vi "Teleop.vi"(10 "Match Info":T1={"Autonomous Elapsed Seconds"=0.0, "TeleOp Elapsed Seconds"=0.0, "Disabled Elapsed Seconds"=0.0, "Visited Autonomous"=FALSE, "Visited TeleOp"=FALSE, "Visited Disabled"=FALSE, "Autonomous Settings"={"Autonomous Style"=enum."Independent", "VI Refnum"=refnum}}, 11 "Call Context":T2) -> ()   [LabVIEW 2015]
doc: "This VI is called for each TeleOp packet received from the DS where the robot is not disabled. It is often used to read from the joysticks and update I/O or to update setpoints for timed control loops. It should complete and return within 20 milliseconds or it may miss DS packets."
uses:
  <vilib>/Rock Robotics/WPI/DriverStation/WPI_DriverStationDerivedRobotMode.ctl
  <vilib>/Rock Robotics/WPI/DriverStation/WPI_DriverStationMatch Info.ctl
  <vilib>/Rock Robotics/WPI/Utilities/WPI_GetSetVariantRefNum.vi
  <vilib>/Rock Robotics/Network Tables/NT Write Boolean Array.vi
  <vilib>/Rock Robotics/Network Tables/NT Write Numeric Array.vi
  <vilib>/Rock Robotics/Network Tables/NT Read Boolean.vi
  <vilib>/Rock Robotics/Network Tables/NT Read Number.vi
  <vilib>/Rock Robotics/WPI/RobotDrive/WPI_RobotDriveArcadeDrive_Standard(NoSaturation).vi
  <vilib>/Rock Robotics/WPI/Ultrasonic/WPI_SonarMB1010AnalogRefNum Registry Get.vi
  <vilib>/Rock Robotics/WPI/Ultrasonic/WPI_SonarMB1010AnalogGetRange.vi
  <vilib>/Rock Robotics/Network Tables/NT Write Number.vi
panel:
  out "Cam Flip":string="Front"
  out "Cam angle\n compensation":dbl=180.0
  out "Drop":dbl=1.0
  out "stuff":dbl
  out "Distance":dbl
  out "Sample Slider 0":dbl(slide) scale=0.0..5.0
  out "Sample Boolean 1":bool
  out "Sample Boolean 0":bool
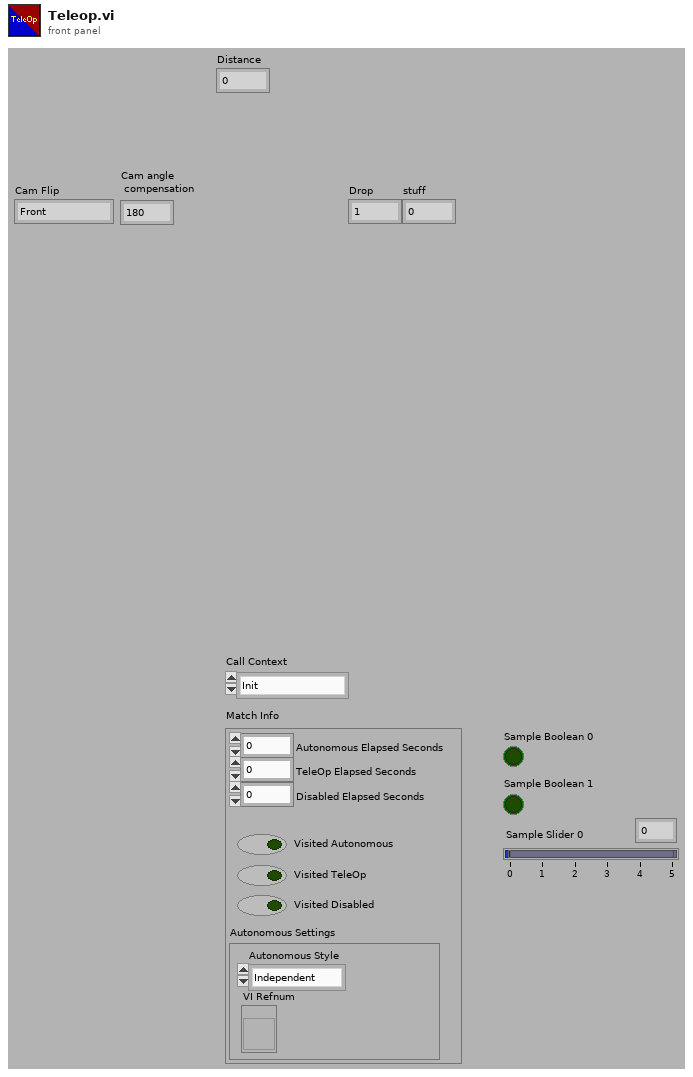
[diagram p1: front panel]
types:
  T1 = typedef "WPI_DriverStationMatch Info.ctl" = cluster{"Autonomous Elapsed Seconds":dbl, "TeleOp Elapsed Seconds":dbl, "Disabled Elapsed Seconds":dbl, "Visited Autonomous":bool, "Visited TeleOp":bool, "Visited Disabled":bool, "Autonomous Settings":cluster{"Autonomous Style":enum16{"Iterative", "Independent"}, "VI Refnum":refnum<vi>}}
  T2 = typedef "WPI_DriverStationDerivedRobotMode.ctl" = enum16{"Init", "Execute", "Stop"}
  T3 = typedef "WPI_JoystickDevRef.ctl" = cluster{"Device":T4}
  T4 = typedef "WPI_JoystickDeviceEnum.ctl" = enum16{"USB 0", "USB 1", "USB 2", "USB 3", "USB 4", "USB 5"}
  T5 = cluster{"Buttons[0]":bool, "Buttons[1]":bool, "Buttons[2]":bool, "Buttons[3]":bool, "Buttons[4]":bool, "Buttons[5]":bool, "Buttons[6]":bool, "Buttons[7]":bool, "Buttons[8]":bool}
  T6 = typedef "WPI_RobotDriveDevRef.ctl" = cluster{"DevStatus":errorcluster, "Motors[]":T7[], "Square Inputs":bool, "Max Output":dbl}
  T7 = typedef "WPI_MotorControlDeviceRef.ctl" = cluster{"DeviceStatus":errorcluster, "Type":T8, "PWM":cluster{"PWM Channel":T9, "DeadBand":T10}, "CAN":cluster{"Device Number":u8, "Control Mode":T11, "Semaphore":T12, "Max Vout":dbl, "TalonSRX Control Mode":T13}, "Invert":bool}
  T8 = typedef "WPI_MotorControlType.ctl" = enum16{"PWM", "CAN", "CANTalonSRX"}
  T9 = typedef "FPGA_DIOPWMChannel.ctl" = enum8{"PWM 0", "PWM 1", "PWM 2", "PWM 3", "PWM 4", "PWM 5", "PWM 6", "PWM 7", "PWM 8", "PWM 9", "PWM MXP 0", "PWM MXP 1", "PWM MXP 2", "PWM MXP 3", "PWM MXP 4", "PWM MXP 5", "PWM MXP 6", "PWM MXP 7", "PWM MXP 8", "PWM MXP 9", "Invalid"}
  T10 = typedef "WPI_PWMDeadband.ctl" = cluster{"Name":string, "maxPositivePwm":i32, "minPositivePwm":i32, "centerPwm":i32, "maxNegativePwm":i32, "minNegativePwm":i32, "angularRange":u16}
  T11 = typedef "WPI_CANJaguar_ControlMode.ctl" = enum8{"Percent VBus", "Current", "Speed", "Position", "Voltage"}
  T12 = typedef "Semaphore RefNum" = refnum<k1>
  T13 = typedef "WPI_CANTalonSRX_APIControlMode.ctl" = enum8{"Percent VBus", "Speed", "Position", "Slave", "Unchanged / Invalid", "Voltage Compensation", "Current", "Motion Profile"}
  T14 = typedef "WPI_ServoDeviceRef.ctl" = cluster{"DeviceStatus":errorcluster, "PWM Channel":T9, "DeadBand":T10}
  T15 = typedef "WPI_SonarMB1010AnalogDeviceRef.ctl" = cluster{"AIDeviceRef":T16, "Scaling factor (V/in)":dbl, "Average Bits":u8}
  T16 = typedef "WPI_AnalogChannelDevRef.ctl" = cluster{"DevStatus":errorcluster, "Analog Channel":T17}
  T17 = typedef "FPGA_AIChannel.ctl" = enum8{"AI 0", "AI 1", "AI 2", "AI 3", "AI MXP 0", "AI MXP 1", "AI MXP 2", "AI MXP 3", "Invalid"}
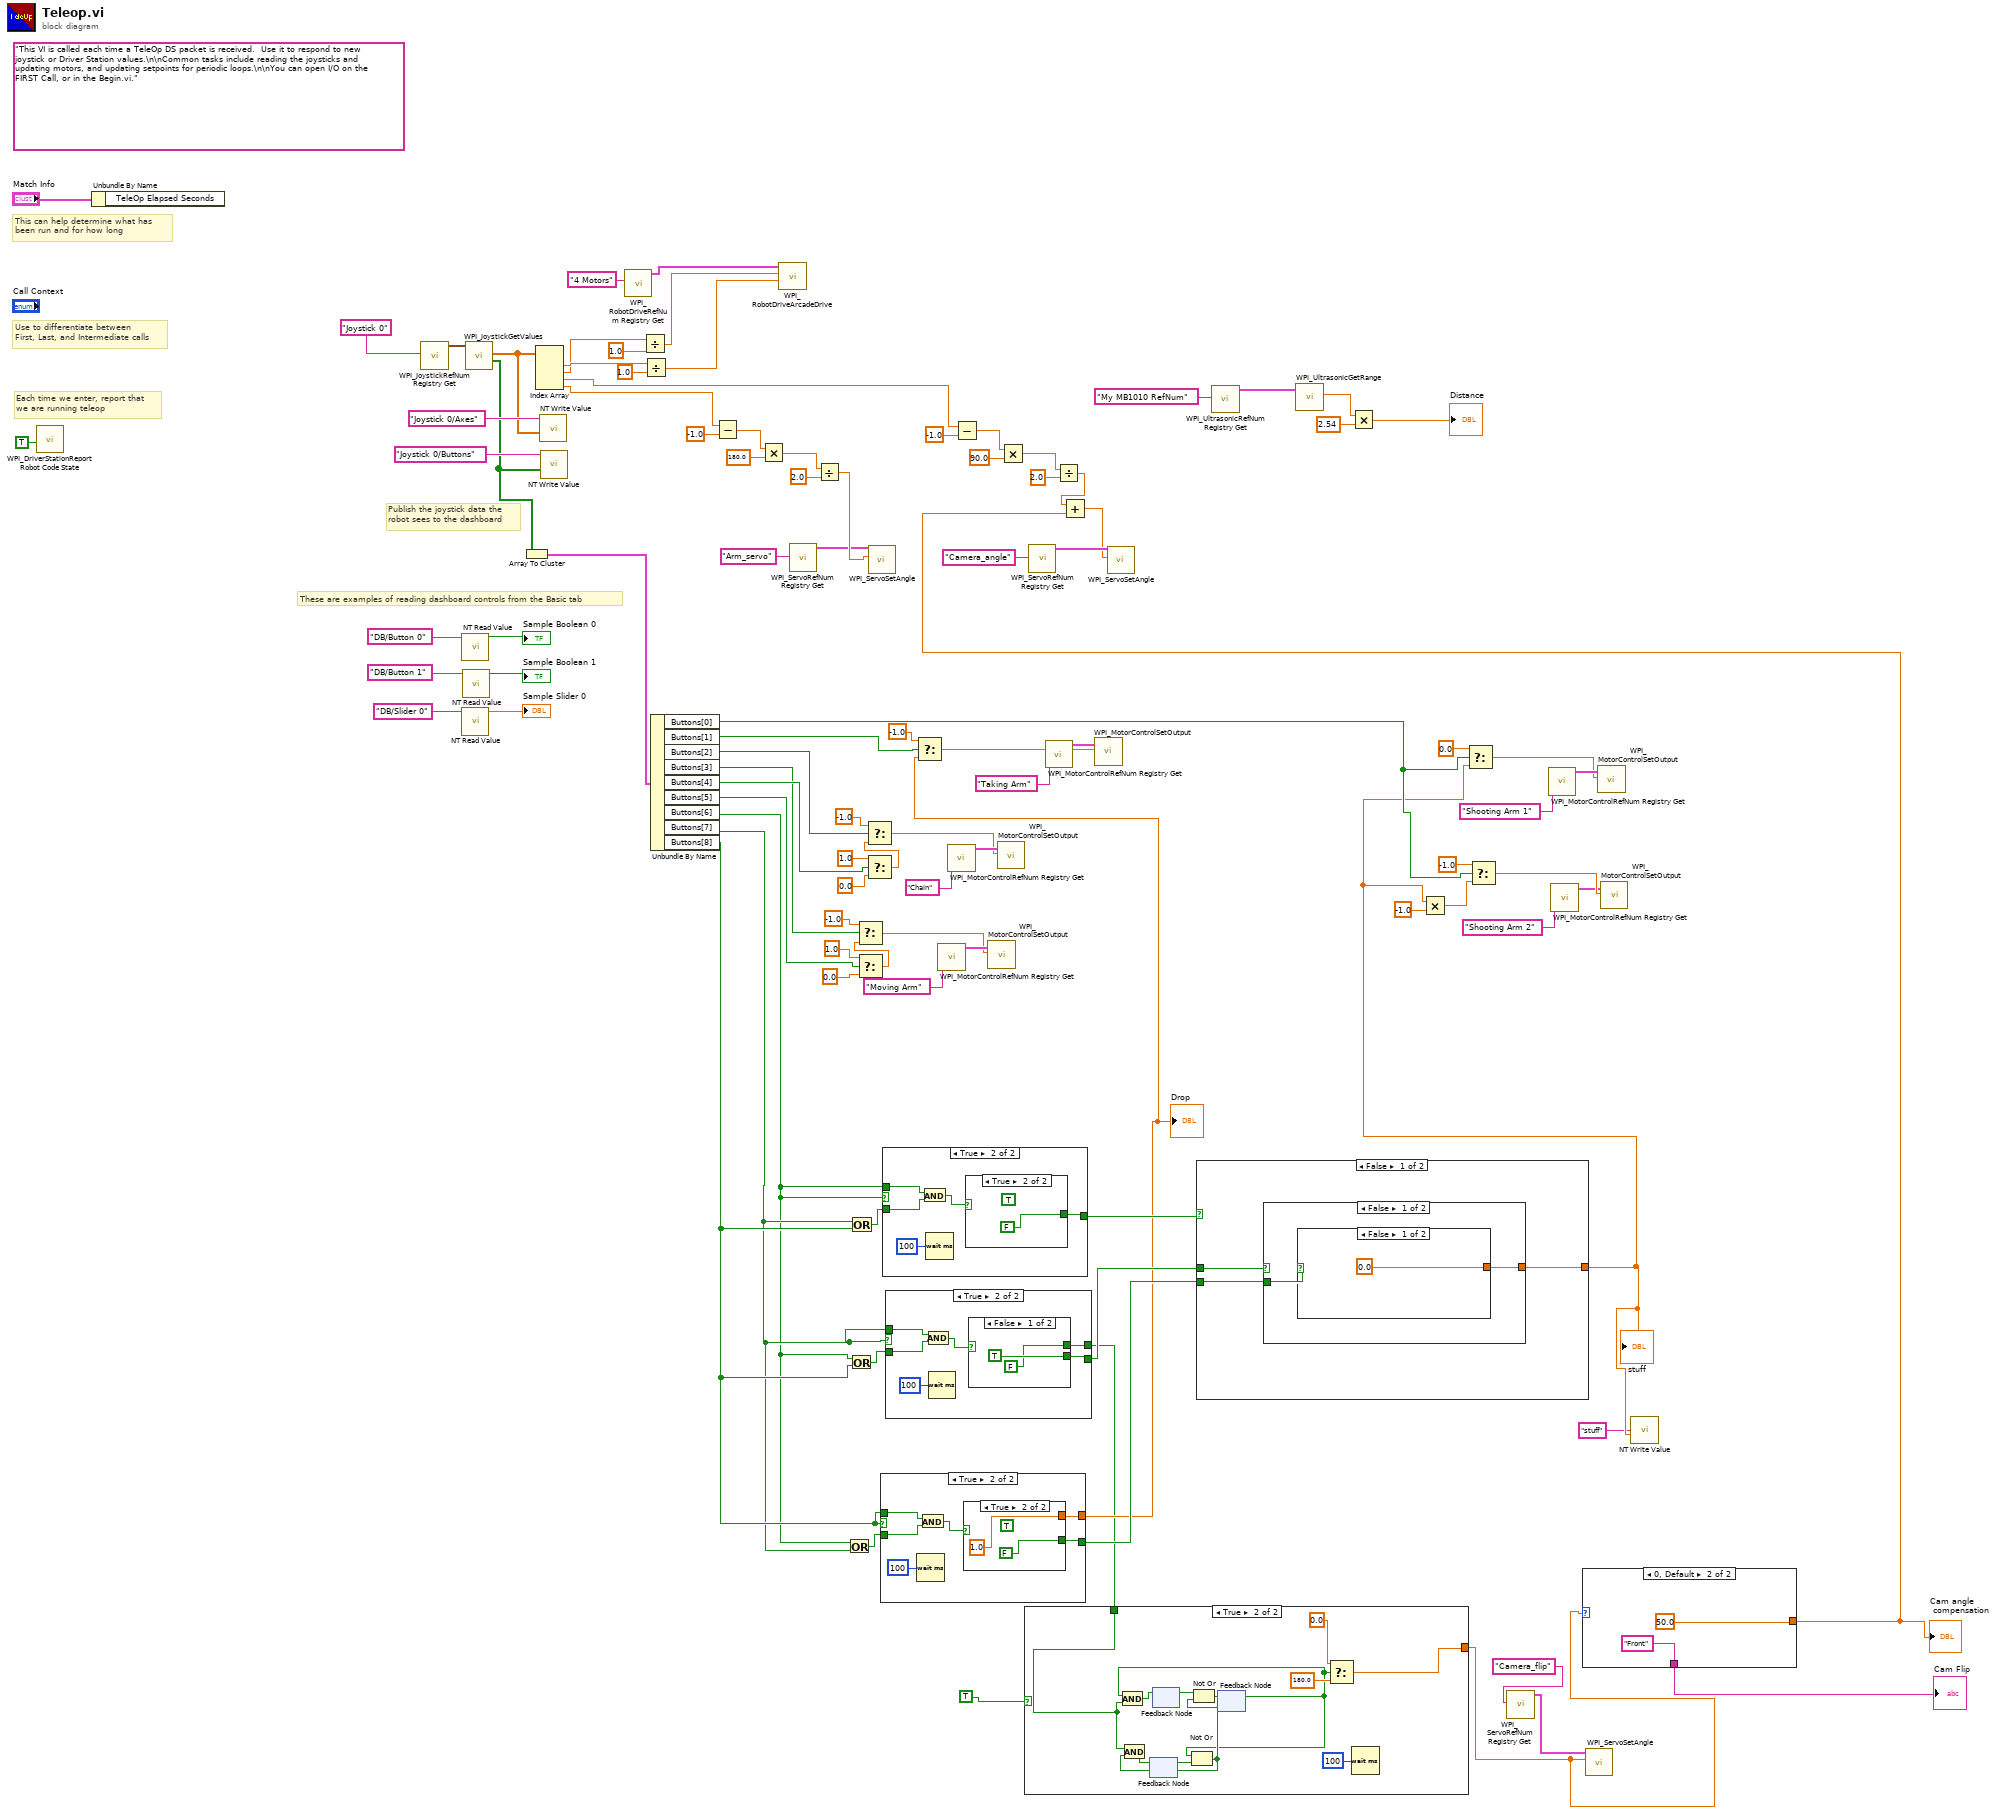
[diagram p0: block diagram]
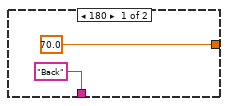
[diagram p2: hidden frame]
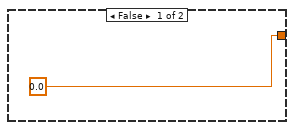
[diagram p3: hidden frame]
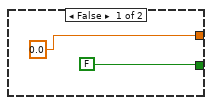
[diagram p4: hidden frame]
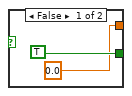
[diagram p5: hidden frame]
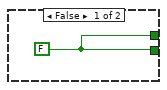
[diagram p6: hidden frame]
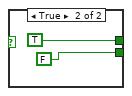
[diagram p7: hidden frame]
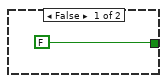
[diagram p8: hidden frame]
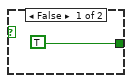
[diagram p9: hidden frame]
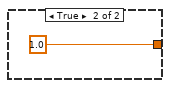
[diagram p10: hidden frame]
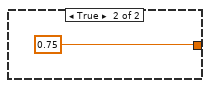
[diagram p11: hidden frame]
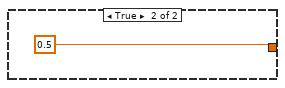
[diagram p12: hidden frame]
diagram:
  (unwired) "This VI is called each time a TeleOp DS packet is received.  Use it to respond to new joystick or Driver Station values.\n\nCommon tasks include reading the joysticks and updating motors, and updating setpoints for periodic loops.\n\nYou can open I/O on the FIRST Call, or in the Begin.vi."
  # "These are examples of reading dashboard controls from the Basic tab"
  # "Publish the joystick data the\nrobot sees to the dashboard"
  # "Each time we enter, report that\nwe are running teleop"
  # "Use to differentiate between\nFirst, Last, and Intermediate calls"
  # "This can help determine what has\nbeen run and for how long"
  n1 = call <vilib>:"WPI_DriverStationReport Robot Code State.vi"("TeleOp"=TRUE ("Autonomous")) -> ()  [unwired: 10 in, 1 out]
  n2 = Unbundle By Name("Match Info") -> ()  [unwired: 1 out]
  n3 = call <vilib>:"WPI_JoystickRefNum Registry Get.vi"("refnum name"="Joystick 0") -> ("JoystickDevRef"=w98:T3)  [unwired: 1 in, 9 out]
  n4 = call-poly <vilib>:"NT Read Value.vi"("Name"="DB/Button 0" ("refnum name")) -> ("Boolean"=→"Sample Boolean 0":bool)  [unwired: 9 in, 1 out]
  n5 = call-poly <vilib>:"NT Read Value.vi"("Name"="DB/Slider 0" ("refnum name")) -> ("Numeric"=→"Sample Slider 0":dbl)  [unwired: 9 in, 1 out]
  n6 = call-poly <vilib>:"NT Read Value.vi"("Name"="DB/Button 1" ("refnum name")) -> ("Boolean"=→"Sample Boolean 1":bool)  [unwired: 9 in, 1 out]
  n7 = call <vilib>:"WPI_JoystickGetValues.vi"("JoystickDevRef"=w98) -> ("Buttons"=w88:bool[], "Axes"=w87:dbl[])  [unwired: 6 in, 3 out]
  n8 = Array To Cluster(array=w88) -> (cluster=w42:T5)
  n9 = Index Array(array=w87) -> (element #1=w84:dbl, element #2=w83:dbl, element #3=w8:dbl, element #4=w16:dbl)  [unwired: 4 in]
  n10 = call-poly <vilib>:"NT Write Value.vi"("Numeric Array"=w87, "Name"="Joystick 0/Axes") -> ()  [unwired: 9 in, 1 out]
  n11 = call-poly <vilib>:"NT Write Value.vi"("Boolean Array"=w88, "Name"="Joystick 0/Buttons") -> ()  [unwired: 9 in, 1 out]
  n12 = call <vilib>:"WPI_RobotDriveRefNum Registry Get.vi"("refnum name"="4 Motors") -> ("RobotDriveDevRef"=w85:T6)  [unwired: 9 in, 1 out]
  n13 = Divide(x=w83, y=1.0) -> (x/y=w80:dbl)
  n14 = Divide(x=w84, y=1.0) -> (x/y=w79:dbl)
  n15 = Unbundle By Name "Unbundle By Name"(w42) -> ("Buttons[0]"=w55:bool, "Buttons[1]"=w43:bool, "Buttons[2]"=w47:bool, "Buttons[3]"=w45:bool, "Buttons[4]"=w46:bool, "Buttons[5]"=w44:bool, "Buttons[6]"=w22:bool, "Buttons[7]"=w23:bool, "Buttons[8]"=w25:bool)
  n16 = Subtract(x=w16, y=-1.0) -> (x-y=w35:dbl)
  n17 = Multiply(x=w35, y=180.0) -> (x*y=w37:dbl)
  n18 = call-poly <vilib>:"WPI_RobotDriveArcadeDrive.vi"("Y axis value"=w79, "X axis value"=w80, "RobotDriveDevRef"=w85) -> ()  [unwired: 6 in, 3 out]
  n19 = call <vilib>:"WPI_ServoRefNum Registry Get.vi"("refnum name"="Arm_servo") -> ("ServoDeviceRef"=w31:T14)  [unwired: 9 in, 1 out]
  n20 = Divide(x=w37, y=2.0) -> (x/y=w38:dbl)
  n21 = Or(x=w22, y=w23) -> (x .or. y?=w24:bool)
  n22 = Or(x=w22, y=w25) -> (x .or. y?=w26:bool)
  n23 = Or(x=w23, y=w25) -> (x .or. y?=w27:bool)
  n24 = Select(t=1.0, s=w44, f=0.0) -> (s? t:f=w60:dbl)
  n25 = Select(t=-1.0, s=w45, f=w60) -> (s? t:f=w56:dbl)
  n26 = Select(t=1.0, s=w46, f=0.0) -> (s? t:f=w68:dbl)
  n27 = Select(t=-1.0, s=w47, f=w68) -> (s? t:f=w53:dbl)
  n28 = call <vilib>:"WPI_ServoSetAngle.vi"("Angle"=w38, "ServoDeviceRef"=w31) -> ()  [unwired: 8 in, 2 out]
  n29 = case shown="True" w25 {
    tunnel: w25 -> [_ w108]
    tunnel: w24 -> [_ w107]
    tunnel: [FALSE w105] -> w28
    tunnel: [0.0 w104] -> w21
    frame False {
    }
    frame True {
      n30 = Wait (ms)(milliseconds to wait=u32 100) -> ()  [unwired: 1 out]
      n31 = And(x=w108, y=w107) -> (x .and. y?=w106:bool)
      n32 = case shown="True" w106 {
        tunnel: [TRUE FALSE] -> w105
        tunnel: [0.0 1.0] -> w104
        frame False {
        }
        frame True {
          (unwired) TRUE
        }
      }
    }
  }
  "Drop" <- w21
  n33 = case shown="True" w22 {
    tunnel: w22 -> [_ w118]
    tunnel: w27 -> [_ w117]
    tunnel: [FALSE w115] -> w30
    frame False {
    }
    frame True {
      n34 = And(x=w118, y=w117) -> (x .and. y?=w116:bool)
      n35 = Wait (ms)(milliseconds to wait=u32 100) -> ()  [unwired: 1 out]
      n36 = case shown="True" w116 {
        tunnel: [TRUE FALSE] -> w115
        frame False {
        }
        frame True {
          (unwired) TRUE
        }
      }
    }
  }
  n37 = case shown="True" w23 {
    tunnel: w23 -> [_ w127]
    tunnel: w26 -> [_ w126]
    tunnel: [w121 w124] -> w29
    tunnel: [w121 w123] -> w20
    frame False {
      w121 = FALSE
    }
    frame True {
      n38 = And(x=w127, y=w126) -> (x .and. y?=w125:bool)
      n39 = Wait (ms)(milliseconds to wait=u32 100) -> ()  [unwired: 1 out]
      n40 = case shown="False" w125 {
        tunnel: [TRUE FALSE] -> w124
        tunnel: [FALSE TRUE] -> w123
        frame False {
        }
        frame True {
        }
      }
    }
  }
  n41 = Select(t=-1.0, s=w43, f=w21) -> (s? t:f=w72:dbl)
  n42 = call <vilib>:"WPI_MotorControlRefNum Registry Get.vi"("refnum name"="Moving Arm") -> ("MotorControlDevRef"=w61:T7)  [unwired: 9 in, 1 out]
  n43 = call <vilib>:"WPI_MotorControlRefNum Registry Get.vi"("refnum name"="Chain") -> ("MotorControlDevRef"=w67:T7)  [unwired: 9 in, 1 out]
  n44 = Subtract(x=w8, y=-1.0) -> (x-y=w13:dbl)
  n45 = call <vilib>:"WPI_MotorControlSetOutput.vi"("Output"=w56, "MotorControlDevRef"=w61) -> ()  [unwired: 7 in, 3 out]
  n46 = call <vilib>:"WPI_MotorControlSetOutput.vi"("Output"=w53, "MotorControlDevRef"=w67) -> ()  [unwired: 7 in, 3 out]
  n47 = Multiply(x=w13, y=90.0) -> (x*y=w15:dbl)
  n48 = case shown="True" TRUE {
    tunnel: w20 -> [_ w142]
    tunnel: [0.0 w133] -> w5
    frame False {
    }
    frame True {
      n49 = feedback #1() -> (w137:bool)  [unwired: 1 in]
      n50 = feedback #2() -> (w140:bool)  [unwired: 1 in]
      n51 = feedback #3() -> (w135:bool)  [unwired: 1 in]
      n52 = And(x=w135, y=w142) -> (x .and. y?=w141:bool)
      n53 = feedback-in #2(w141) -> ()
      n54 = Not Or(1:w137, 2:w135) -> (0:w139:bool)
      n55 = And(x=w142, y=w139) -> (x .and. y?=w138:bool)
      n56 = feedback-in #1(w138) -> ()
      n57 = Not Or(1:w139, 2:w140) -> (0:w136:bool)
      n58 = feedback-in #3(w136) -> ()
      n59 = Select(t=0.0, s=w135, f=180.0) -> (s? t:f=w133:dbl)
      n60 = Wait (ms)(milliseconds to wait=u32 100) -> ()  [unwired: 1 out]
    }
  }
  n61 = call <vilib>:"WPI_ServoRefNum Registry Get.vi"("refnum name"="Camera_angle") -> ("ServoDeviceRef"=w9:T14)  [unwired: 9 in, 1 out]
  n62 = call <vilib>:"WPI_MotorControlRefNum Registry Get.vi"("refnum name"="Taking Arm") -> ("MotorControlDevRef"=w74:T7)  [unwired: 9 in, 1 out]
  n63 = Divide(x=w15, y=2.0) -> (x/y=w6:dbl)
  n64 = call <vilib>:"WPI_MotorControlSetOutput.vi"("Output"=w72, "MotorControlDevRef"=w74) -> ()  [unwired: 7 in, 3 out]
  n65 = case shown="False" w30 {
    tunnel: w29 -> [w147 _]
    tunnel: w28 -> [w146 _]
    tunnel: [w145 0.5] -> w2
    frame False {
      n66 = case shown="False" w147 {
        tunnel: w146 -> [w149 _]
        tunnel: [w148 0.75] -> w145
        frame False {
          n67 = case shown="False" w149 {
            tunnel: [0.0 1.0] -> w148
            frame False {
            }
            frame True {
            }
          }
        }
        frame True {
        }
      }
    }
    frame True {
    }
  }
  "stuff" <- w2
  n68 = call-poly <vilib>:"WPI_UltrasonicRefNum Registry Get.vi"("refnum name"="My MB1010 RefNum") -> ("SonarMB1010AnalogDevRef"=w50:T15)  [unwired: 9 in, 1 out]
  n69 = call-poly <vilib>:"WPI_UltrasonicGetRange.vi"("SonarMB1010AnalogDevRef"=w50) -> ("Distance"=w51:dbl)  [unwired: 8 in, 2 out]
  n70 = Multiply(x=w51, y=2.54) -> (x*y=→"Distance":dbl)
  n71 = Multiply(x=w2, y=-1.0) -> (x*y=w40:dbl)
  n72 = Select(t=0.0, s=w55, f=w2) -> (s? t:f=w54:dbl)
  n73 = Select(t=-1.0, s=w55, f=w40) -> (s? t:f=w77:dbl)
  n74 = call <vilib>:"WPI_ServoRefNum Registry Get.vi"("refnum name"="Camera_flip") -> ("ServoDeviceRef"=w18:T14)  [unwired: 9 in, 1 out]
  n75 = call <vilib>:"WPI_MotorControlRefNum Registry Get.vi"("refnum name"="Shooting Arm 1") -> ("MotorControlDevRef"=w78:T7)  [unwired: 9 in, 1 out]
  n76 = call <vilib>:"WPI_MotorControlRefNum Registry Get.vi"("refnum name"="Shooting Arm 2") -> ("MotorControlDevRef"=w75:T7)  [unwired: 9 in, 1 out]
  n77 = case shown="0, Default" w5 {
    tunnel: [70.0 50.0] -> w4
    tunnel: ["Back" "Front"] -> w3
    frame 180 {
    }
    frame 0, Default {
    }
  }
  "Cam angle\n compensation" <- w4
  "Cam Flip" <- w3
  n78 = Add(x=w6, y=w4) -> (x+y=w7:dbl)
  n79 = call <vilib>:"WPI_ServoSetAngle.vi"("Angle"=w7, "ServoDeviceRef"=w9) -> ()  [unwired: 8 in, 2 out]
  n80 = call <vilib>:"WPI_ServoSetAngle.vi"("Angle"=w5, "ServoDeviceRef"=w18) -> ()  [unwired: 8 in, 2 out]
  n81 = call <vilib>:"WPI_MotorControlSetOutput.vi"("Output"=w54, "MotorControlDevRef"=w78) -> ()  [unwired: 7 in, 3 out]
  n82 = call <vilib>:"WPI_MotorControlSetOutput.vi"("Output"=w77, "MotorControlDevRef"=w75) -> ()  [unwired: 7 in, 3 out]
  n83 = call-poly <vilib>:"NT Write Value.vi"("Numeric"=w2, "Name"="stuff") -> ()  [unwired: 9 in, 1 out]
